vi "Write Synch.vi"(8 "error in":errorcluster, 10 "Timing":T1={"Source"="", "Sample Rate (10k)"=10000.0, "sample mode"=10178, "samples per channel"=1000} {"sample mode" items=["Finite Samples"=10178, "Continuous Samples"=10123, "Hardware Timed Single Point"=12522]}, 11 "AnalogInput in":refnum<class "AnalogInput.lvclass">) -> (0 "error out":errorcluster, 3 "AnalogInput out":refnum<class "AnalogInput.lvclass">)   [LabVIEW 2019, in "AnalogInput.lvlib" / "AnalogInput.lvclass"]
uses:
  Library/AnalogInput.lvclass
  Custom Controls/Synch Settings.ctl
  Library/AnalogInput.lvclass/AnalogInput.ctl
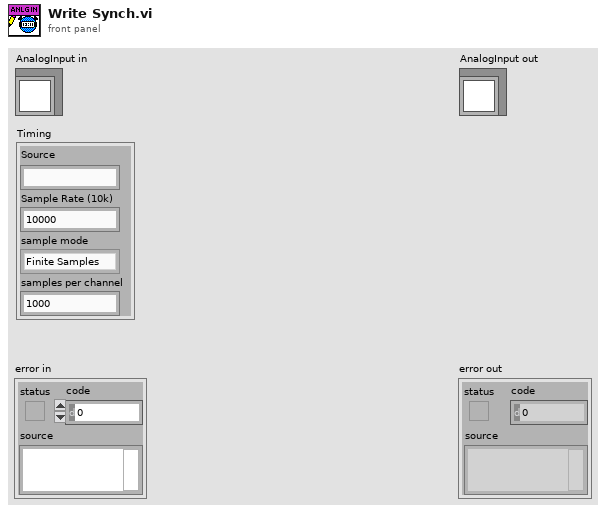
[diagram p1: front panel]
types:
  T1 = typedef "AnalogInput.lvlib/AnalogInput.lvclass/Synch Settings.ctl" = cluster{"Source":string, "Sample Rate (10k)":dbl, "sample mode":i32, "samples per channel":i32}
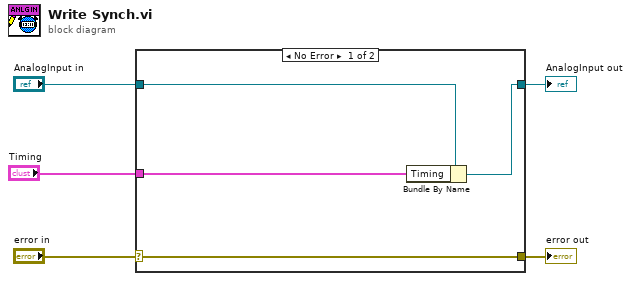
[diagram p0: block diagram]
diagram:
  n1 = case shown="No Error" "error in" {
    selector: "error in" -> [w9 w10]
    tunnel: [w9 w10] -> w4
    tunnel: [w7 w11] -> w2
    tunnel: "AnalogInput in" -> [w8 w11]
    tunnel: "Timing" -> [w6 _]
    frame No Error {
      n2 = Bundle By Name(cluster=w8, "Timing"=w6) -> (w7:refnum<class "AnalogInput.lvclass">)
    }
    frame Error {
    }
  }
  "error out" <- w4
  "AnalogInput out" <- w2
